vi "Renishaw-XL80_GetEC10Version.vi"(8 "error in (no error)":errorcluster, 11 "Renishaw-XL80 in":refnum<class "Renishaw-XL80.lvclass">) -> (0 "error out":errorcluster, 2 "EC10Version":string, 3 "Renishaw-XL80 out":refnum<class "Renishaw-XL80.lvclass">)   [LabVIEW 2024, in "Renishaw-XL80.lvclass"]
doc: "This read only property returns the version string of the EC10.\n\nDefinition\nHRESULTget_EC10Version( [out, retval] BSTR* pVal);\nParameters\npVal\nA variable that will be set to the version string of the EC10.\n\nComments\nThis property will return with an HRESULT of E_FAIL if the client has not previously connected to a DX10 by calling Connect.\n\nThe property will normally return an HRESULT of S_OK. However, it will return E_POINTER if the client supplies a null pointer for pVal, and in extremely low memory conditions it will return E_NOMEMORY.\n\nNote: if there is a XL laser connected to the DX10Adaptor COM interface this property will return the firmare version of the associated XC compensator."
uses:
  Renishaw-XL80.lvclass
  Renishaw-XL80.lvclass/Renishaw-XL80.ctl
  D:/A.C.M/Example CSharp_64/bin/Debug/Interop.DX10SDKADAPTORLib.dll
  Example CSharp_64/bin/Debug/Interop.DX10SDKADAPTORLib.dll
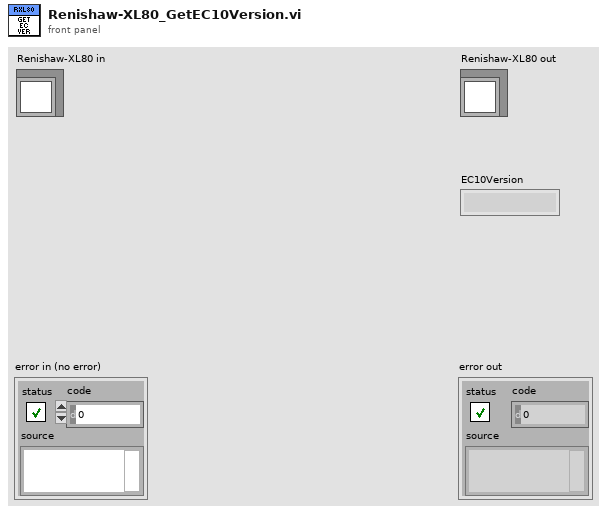
[diagram p1: front panel]
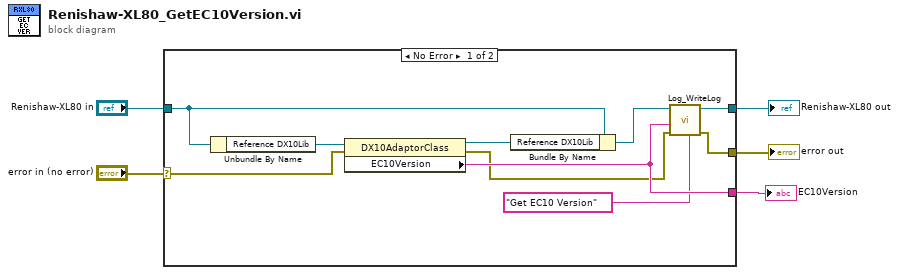
[diagram p0: block diagram]
diagram:
  n1 = case shown="No Error" "error in (no error)" {
    selector: "error in (no error)" -> [w12 w17]
    tunnel: [w7 w17] -> w4
    tunnel: [w10 w16] -> w2
    tunnel: "Renishaw-XL80 in" -> [w13 w16]
    tunnel: [w9 _] -> w1
    frame No Error {
      n2 = Unbundle By Name(w13) -> ("Reference DX10Lib"=w15:refnum<k24>)
      n3 = property class="DX10AdaptorClass"(reference=w15, error in=w12) -> (reference out=w14:refnum<k24>, error out=w8:errorcluster, "EC10Version"=w9:string)
      n4 = Bundle By Name(cluster=w13, "Reference DX10Lib"=w14) -> (w11:refnum<class "Renishaw-XL80.lvclass">)
      n5 = call-dynamic "Log_WriteLog.vi"("Additional text"="Get EC10 Version", "error in (no error)"=w8, "Response"=w9, "Log in"=w11) -> ("error out"=w7:errorcluster, "Log out"=w10:refnum<class "Renishaw-XL80.lvclass">)  [unwired: 6 in]
    }
    frame Error {
    }
  }
  "error out" <- w4
  "Renishaw-XL80 out" <- w2
  "EC10Version" <- w1
